vi "REV2_Write_Config.vi"(7 "ID":u8, 8 "error in (no error)":errorcluster, 9 "Data":dbl[](array[numeric]), 10 "Config Addr":T1[](array[typedef]) items=["ID", "Mode", "Baudrate", "Homing Offset", "Id P gain", "Id I gain", "Id D gain", "Iq P gain", "Iq I gain", "Iq D gain", "Velo P gain", "Velo I gain", "Velo D gain", "Posi P gain", "Posi I gain", "Posi D gain", "DirectForce P", "DirectForce I", "DirectForce D", "Limit Id Max", "Limit Iq Max", "Limit Velo Max", "Limit Posi Min", "Limit Posi Max", "Voltage Min", "Voltage Max", "Watchdog", "Temperature Low", "Temperature High"], 11 "VISA Refnum in":refnum<visa-resource-name>) -> (0 "error out":errorcluster, 3 "VISA Refnum out":refnum<visa-resource-name>)   [LabVIEW 2016, in "REV_2.lvlib"]
uses:
  REV_2.lvlib
  REV2_Instructions.ctl
  REV2_Config_Addr.ctl
panel:
  out "Output":string
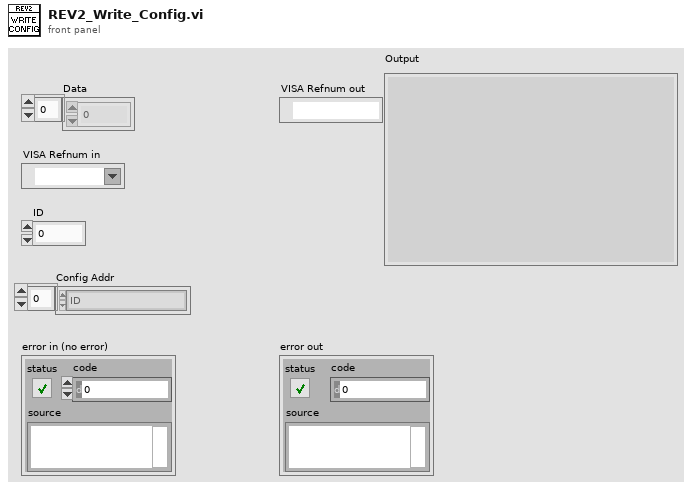
[diagram p1: front panel]
types:
  T1 = typedef "REV_2.lvlib/REV2_Config_Addr.ctl" = u8
  T2 = enum16{"big-endian, network order", "native, host order", "little-endian"}
  T3 = typedef "REV_2.lvlib/REV2_Instructions.ctl" = u8
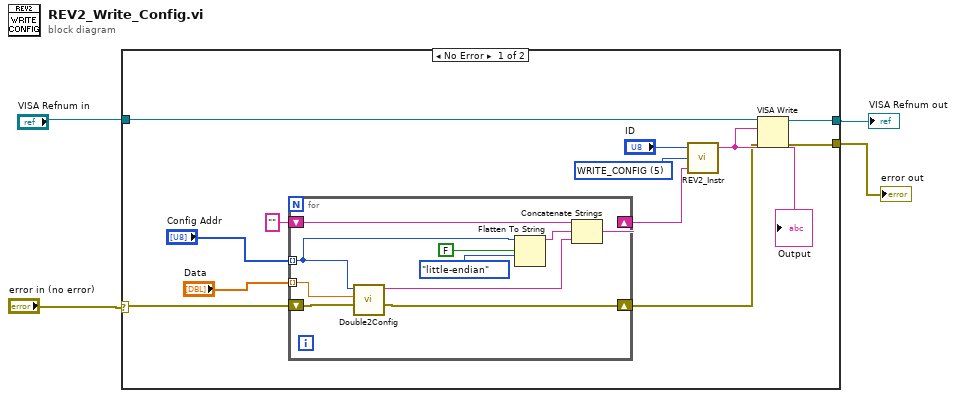
[diagram p0: block diagram]
diagram:
  n1 = case shown="No Error" "error in (no error)" {
    selector: "error in (no error)" -> [w5 w28]
    tunnel: [w11 w27] -> w4
    tunnel: [w10 w28] -> w3
    tunnel: "VISA Refnum in" -> [w7 w27]
    frame No Error {
      w15 = T3 5 items=["PING"=1, "READ_STAT"=2, "WRITE_STAT"=3, "READ_CONFIG"=4, "WRITE_CONFIG"=5, "SAVE_CONFIG"=6] ("Instruction")
      n2 = for {
        tunnel: "Config Addr" -> [w20] mode=indexing
        tunnel: "Data" -> [w19] mode=indexing
        shift-right: [w21] -> w14
        shift-left: "" -> [w22]
        shift-right: [w17] -> w6
        shift-left: w5 -> [w18]
        n3 = call "Double2Config.vi"("error in (no error)"=w18, "Data"=w19, "Config Address"=w20) -> ("error out"=w17:errorcluster, "data string"=w23:string)  [unwired: 7 in]
        n4 = Flatten To String(anything=w20, prepend array or string size? (T)=FALSE, byte order (0:big-endian, network order)=T2."little-endian") -> (data string=w24:string)  [unwired: 1 in, 2 out]
        n5 = Concatenate Strings(w22, w24, w23) -> (w21:string)
      }
      n6 = call "REV2_Instr.vi"("Parameter"=w14, "Instruction"=w15, "ID"="ID") -> ("Output"=w9:string)  [unwired: 2 in]
      "Output" <- w9
      n7 = VISA Write(VISA resource name=w7, write buffer=w9, error in (no error)=w6) -> (VISA resource name out=w11:refnum<visa-resource-name>, error out=w10:errorcluster)  [unwired: 1 out]
    }
    frame Error {
    }
  }
  "VISA Refnum out" <- w4
  "error out" <- w3
